vi "Test Read.vi"   [LabVIEW 2017]
uses:
  <vilib>/Rock Robotics/WPI/SafetyOutput/WPI_SafetyOutputConfigMenu.ctl
  Public/Documents/Cross The Road Electronics/Phoenix-LabVIEW/Motor Controller/Controls/CTRE_Phoenix_MotorControl_FeedbackDevice.ctl
  <vilib>/Rock Robotics/WPI/ThirdParty/Phoenix-LabVIEW/Motor Controller/Get/CTRE_Phoenix_MotorController_GetSelectedSensorData.vi
  <vilib>/Rock Robotics/Network Tables/NT Write String.vi
  <vilib>/Rock Robotics/Network Tables/NT Write Number.vi
  SwerveLibrary/Huskie Swerve.lvlib
types:
  T1 = typedef "CTRE_Phoenix_MotorControl_FeedbackDevice.ctl" = i8
  T2 = typedef "WPI_SafetyOutputConfigMenu.ctl" = enum16{"Enable", "Disable"}
  T3 = typedef "WPI_MotorControlDeviceRef.ctl" = cluster{"DeviceStatus":errorcluster, "Type":T4, "PWM":cluster{"PWM Channel":T5, "DeadBand":T6}, "CAN":cluster{"Device Number":u8, "SetOutput VI Ref":variant, "GetOutput VI Ref":variant, "Enable VI Ref":variant, "Disable VI Ref":variant, "Data":variant}, "Invert":bool, "DIO PWM":cluster{"PWM \"Enable\" Channel":T5, "DIOChannel":T7, "PWM Rate":dbl}}
  T4 = typedef "WPI_MotorControlType.ctl" = enum16{"PWM", "CAN", "DIO PWM"}
  T5 = typedef "FPGA_DIOPWMChannel.ctl" = enum8{"PWM 0", "PWM 1", "PWM 2", "PWM 3", "PWM 4", "PWM 5", "PWM 6", "PWM 7", "PWM 8", "PWM 9", "PWM MXP 0", "PWM MXP 1", "PWM MXP 2", "PWM MXP 3", "PWM MXP 4", "PWM MXP 5", "PWM MXP 6", "PWM MXP 7", "PWM MXP 8", "PWM MXP 9", "Invalid"}
  T6 = typedef "WPI_PWMDeadband.ctl" = cluster{"Name":string, "maxPositivePwm":i32, "minPositivePwm":i32, "centerPwm":i32, "maxNegativePwm":i32, "minNegativePwm":i32, "angularRange":u16}
  T7 = typedef "FPGA_DIOChannel.ctl" = enum8{"DIO 0", "DIO 1", "DIO 2", "DIO 3", "DIO 4", "DIO 5", "DIO 6", "DIO 7", "DIO 8", "DIO 9", "DIO MXP 0", "DIO MXP 1", "DIO MXP 2", "DIO MXP 3", "DIO MXP 4", "DIO MXP 5", "DIO MXP 6", "DIO MXP 7", "DIO MXP 8", "DIO MXP 9", "DIO MXP 10", "DIO MXP 11", "DIO MXP 12", "DIO MXP 13", "DIO MXP 14", "DIO MXP 15", "SPI Port CS1", "SPI Port CS2", "SPI Port CS3", "SPI Port MISO", "SPI Port MOSI", "Invalid"}
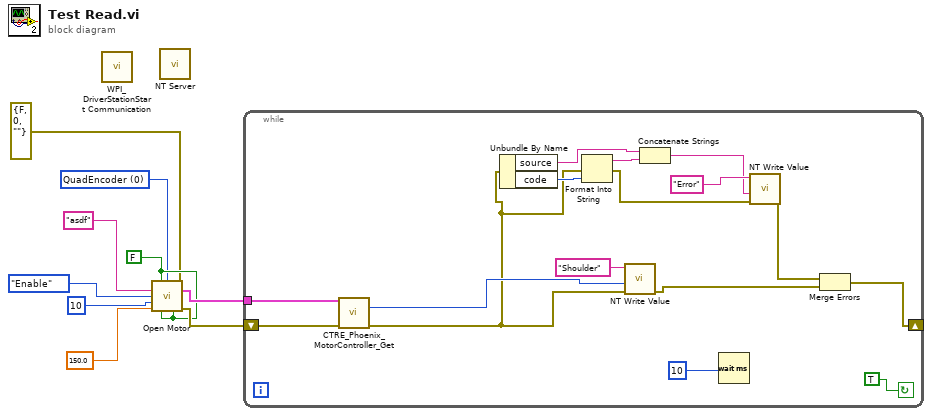
[diagram p0: block diagram]
diagram:
  w2 = T1 0 items=["None"=-1, "QuadEncoder"=0, "Analog"=2, "Tachometer"=4, "Pulse Width Encoded Position"=8, "Sensor Sum (S0 + S1)"=9, "Sensor Difference (D0 - D1)"=10, "Remote Source 0"=11, "Remote Source 1"=12, "Software Emulated"=15] ("Feedback Reference")
  w3 = FALSE ("PID?")
  n1 = call <vilib>:"WPI_DriverStationStart Communication.vi"() -> ()  [unwired: 12 in]
  n2 = call "Open Motor.vi"("PID?"=w3, "Feedback Reference"=w2, "error in"=errorcluster {"status"=FALSE, "code"=0, "source"=""} ("error constant"), "refnum name"="asdf", "mode (safety config)"=WPI_SafetyOutputConfigMenu."Enable", "CAN Device Number"=u8 10 ("Device Number"), "Set sensor position"=150.0, "Reverse Feedback Sensor"=w3, "Invert Power"=w3) -> ("CAN Talon SRX Ref"=w7:T3, "error out"=w8:errorcluster)  [unwired: 5 in]
  n3 = call <vilib>:"NT Server.vi"() -> ()  [unwired: 12 in]
  n4 = while {
    tunnel: w7 -> [w25]
    shift-right: [w13] -> _
    shift-left: w8 -> [w24]
    stop <- TRUE continue-if-true
    n5 = call-poly "CTRE_Phoenix_MotorController_Get.vi"("PhoenixMotorControlDevRef"=w25, "error in"=w24) -> ("Position (Raw Sensor Units)"=w16:i32, "error out"=w15:errorcluster)  [unwired: 10 in, 2 out]
    n6 = Unbundle By Name(w15) -> ("source"=w18:string, "code"=w20:i32)
    n7 = Format Into String(error in=w15, w20) -> (resulting string=w19:string, error out=w14:errorcluster)  [unwired: 2 in]
    n8 = call-poly <vilib>:"NT Write Value.vi"("error in"=w15, "Numeric"=w16, "Name"="Shoulder") -> ("error out"=w11:errorcluster)  [unwired: 8 in]
    n9 = Concatenate Strings(w18, w19) -> (w17:string)
    n10 = Wait (ms)(milliseconds to wait=10) -> ()  [unwired: 1 out]
    n11 = call-poly <vilib>:"NT Write Value.vi"("error in"=w14, "String"=w17, "Name"="Error") -> ("error out"=w12:errorcluster)  [unwired: 8 in]
    n12 = Merge Errors(w12, w11) -> (w13:errorcluster)
  }
